vi "Start Module.vi"() -> (0 "error out":errorcluster, 1 "isAlreadyRunning?":bool=TRUE)   [LabVIEW 2014, in "Events Lib.lvlib"]
uses:
  Events Lib.lvlib
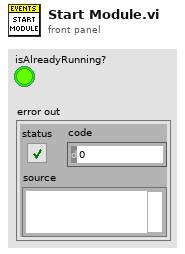
[diagram p1: front panel]
types:
  T1 = enum32{"Bad", "Idle", "Run top level", "Running"}
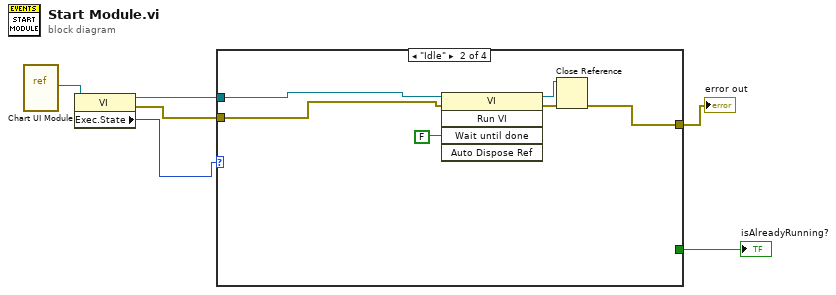
[diagram p0: block diagram]
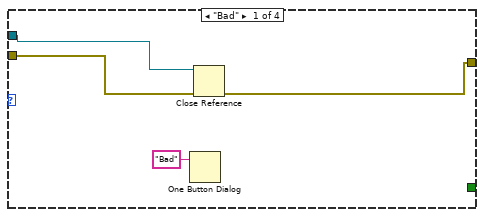
[diagram p2: hidden frame]
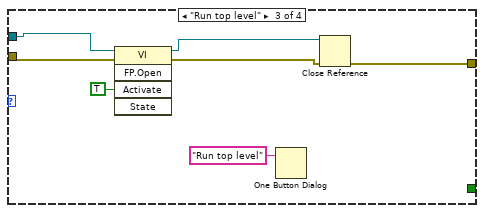
[diagram p3: hidden frame]
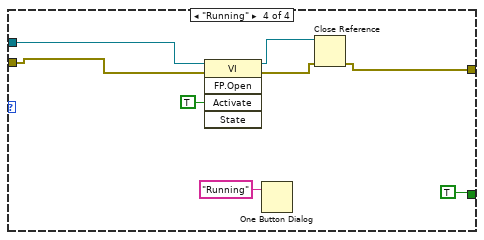
[diagram p4: hidden frame]
diagram:
  n1 = vi-ref "Chart UI Module.vi"() -> (w6:refnum<vi>)
  n2 = property class="VI"(reference=w6) -> (reference out=w4:refnum<vi>, error out=w3:errorcluster, "Exec.State"=w5:T1)  [unwired: 1 in]
  n3 = case shown="\"Idle\"" w5 {
    tunnel: w4 -> [w10 w12 w22 w30]
    tunnel: w3 -> [w8 w11 w21 w29]
    tunnel: [w9 w13 w20 w26] -> w2
    tunnel: [_ _ _ TRUE] -> w1
    frame "Bad" {
      n4 = One Button Dialog(message="Bad") -> ()  [unwired: 1 in, 1 out]
      n5 = Close Reference(reference=w10, error in (no error)=w8) -> (error out=w9:errorcluster)
    }
    frame "Idle" {
      n6 = invoke class="VI" method="Run VI"(reference=w12, error in=w11, "Wait until done"=FALSE ("Wait Until Done")) -> (reference out=w14:refnum<vi>, error out=w15:errorcluster)  [unwired: 2 in, 3 out]
      n7 = Close Reference(reference=w14, error in (no error)=w15) -> (error out=w13:errorcluster)
    }
    frame "Run top level" {
      n8 = invoke class="VI" method="FP.Open"(reference=w22, error in=w21, "Activate"=TRUE ("Activate?")) -> (reference out=w18:refnum<vi>, error out=w19:errorcluster)  [unwired: 2 in, 3 out]
      n9 = One Button Dialog(message="Run top level") -> ()  [unwired: 1 in, 1 out]
      n10 = Close Reference(reference=w18, error in (no error)=w19) -> (error out=w20:errorcluster)
    }
    frame "Running" {
      n11 = invoke class="VI" method="FP.Open"(reference=w30, error in=w29, "Activate"=TRUE ("Activate?")) -> (reference out=w28:refnum<vi>, error out=w27:errorcluster)  [unwired: 2 in, 3 out]
      n12 = One Button Dialog(message="Running") -> ()  [unwired: 1 in, 1 out]
      n13 = Close Reference(reference=w28, error in (no error)=w27) -> (error out=w26:errorcluster)
    }
  }
  "error out" <- w2
  "isAlreadyRunning?" <- w1
